vi "首页.vi"() -> ()   [LabVIEW 2016]
uses:
  <vilib>/Utility/miscctls.llb/LVPointTypeDef.ctl
  <vilib>/Utility/sysdir.llb/System Directory Type.ctl
  <vilib>/addons/database/_DB Variant To Data/Database Variant To Data.xnode
  PLC/PLC.lvlib
panel:
  out "大项目框 17":T1(xcontrol)
  out "大项目框 16":T1(xcontrol)
  out "大项目框 15":T1(xcontrol)
  out "大项目框 14":T1(xcontrol)
  out "大项目框 13":T1(xcontrol)
  in  "左箭头":bool
  in  "右箭头":bool
  out "大项目框 12":T1(xcontrol)
  out "大项目框 11":T1(xcontrol)
  out "大项目框 10":T1(xcontrol)
  out "大项目框 9":T1(xcontrol)
  out "大项目框 8":T1(xcontrol)
  out "大项目框 7":T1(xcontrol)
  out "大项目框 6":T1(xcontrol)
  out "大项目框 5":T1(xcontrol)
  out "大项目框 4":T1(xcontrol)
  out "大项目框 3":T1(xcontrol)
  out "大项目框 2":T1(xcontrol)
  out "大项目框":T1(xcontrol)
  out "湿度":string="75.5 %"
  out "室温":string="25.8 ℃"
  # "室温:"
  # "湿度:"
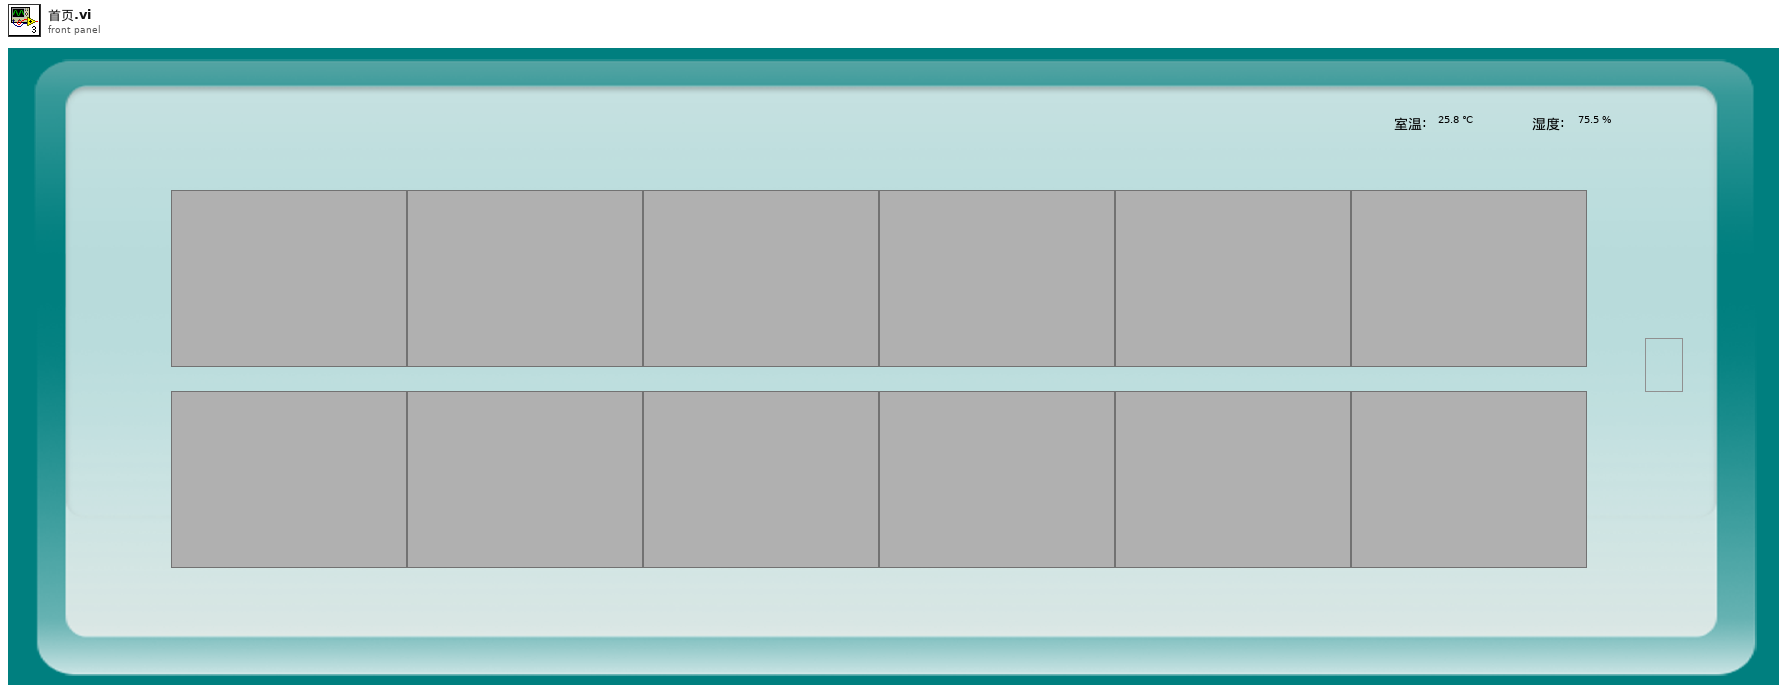
[diagram p1: front panel]
types:
  T1 = cluster{"中文项目名称":string, "英文项目名称":string, "单位":string, "浓度值":string}
  T2 = typedef "LVPointTypeDef.ctl" = cluster{"Horizontal":i16, "Vertical":i16}
  T3 = cluster{"AD0":sgl, "AD1":sgl, "AD2":sgl, "AD3":sgl, "AD4":sgl, "AD5":sgl}
  T4 = typedef "LVDateTimeRec.ctl" = cluster{"秒数的小数部分":dbl, "秒":i32, "分":i32, "时":i32, "日":i32, "月":i32, "年":i32, "天数（周）":i32, "天数（年）":i32, "DST":i32}
  T5 = cluster{"时间标识":timestamp, "监测值":sgl, "单位":string}
  T6 = cluster{"显示参数中文名":string, "显示参数英文名":string, "显示浓度":string, "显示单位":string}[]
  T7 = cluster{"显示参数中文名":string, "显示参数英文名":string, "显示浓度":string, "显示单位":string}
  T8 = typedef "System Directory Type.ctl" = i32
  T9 = cluster{"水温":bool, "pH":bool, "DO":bool, "Cond":bool, "Turb":bool, "氨氮":bool, "总磷":bool, "总氮":bool, "CODMn":bool, "CODCr":bool, "水位":bool, "流速":bool, "瞬时流量":bool, "室温":bool, "湿度":bool, "叶绿素a":bool, "藻密度":bool}
  T10 = cluster{"中文项目名称":string, "英文项目名称":string, "浓度值":string, "单位":string}
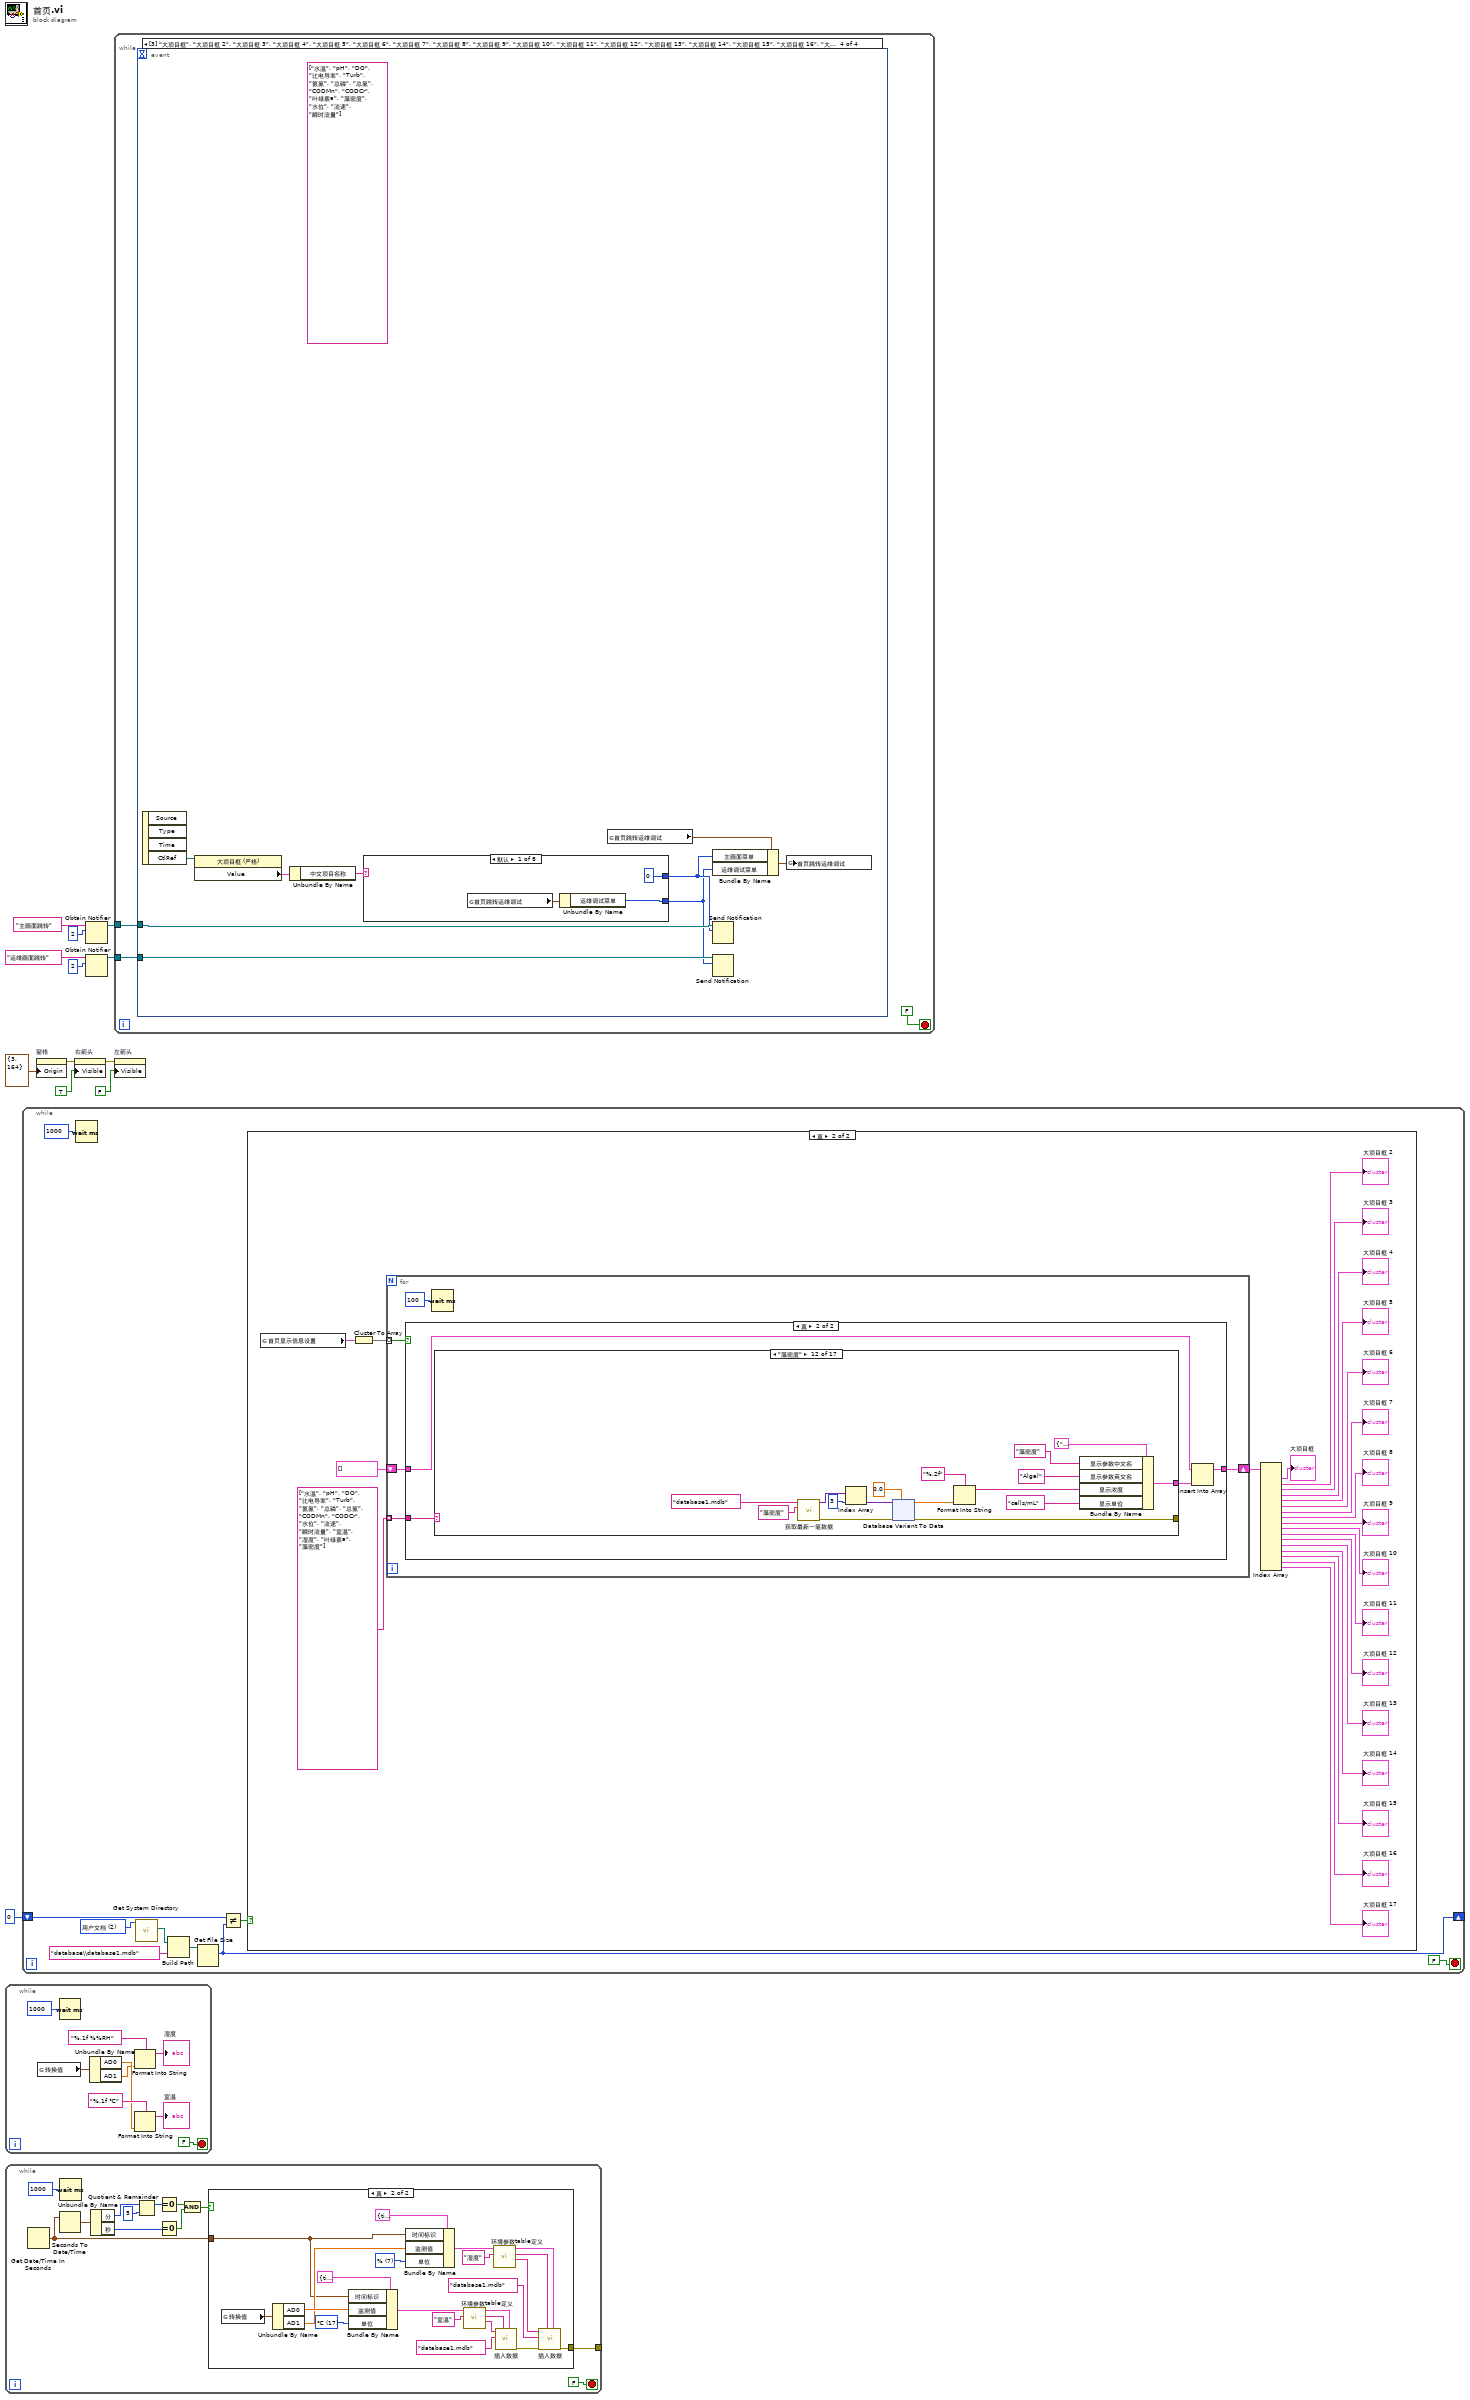
[diagram p0: block diagram]
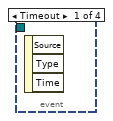
[diagram p3: hidden frame]
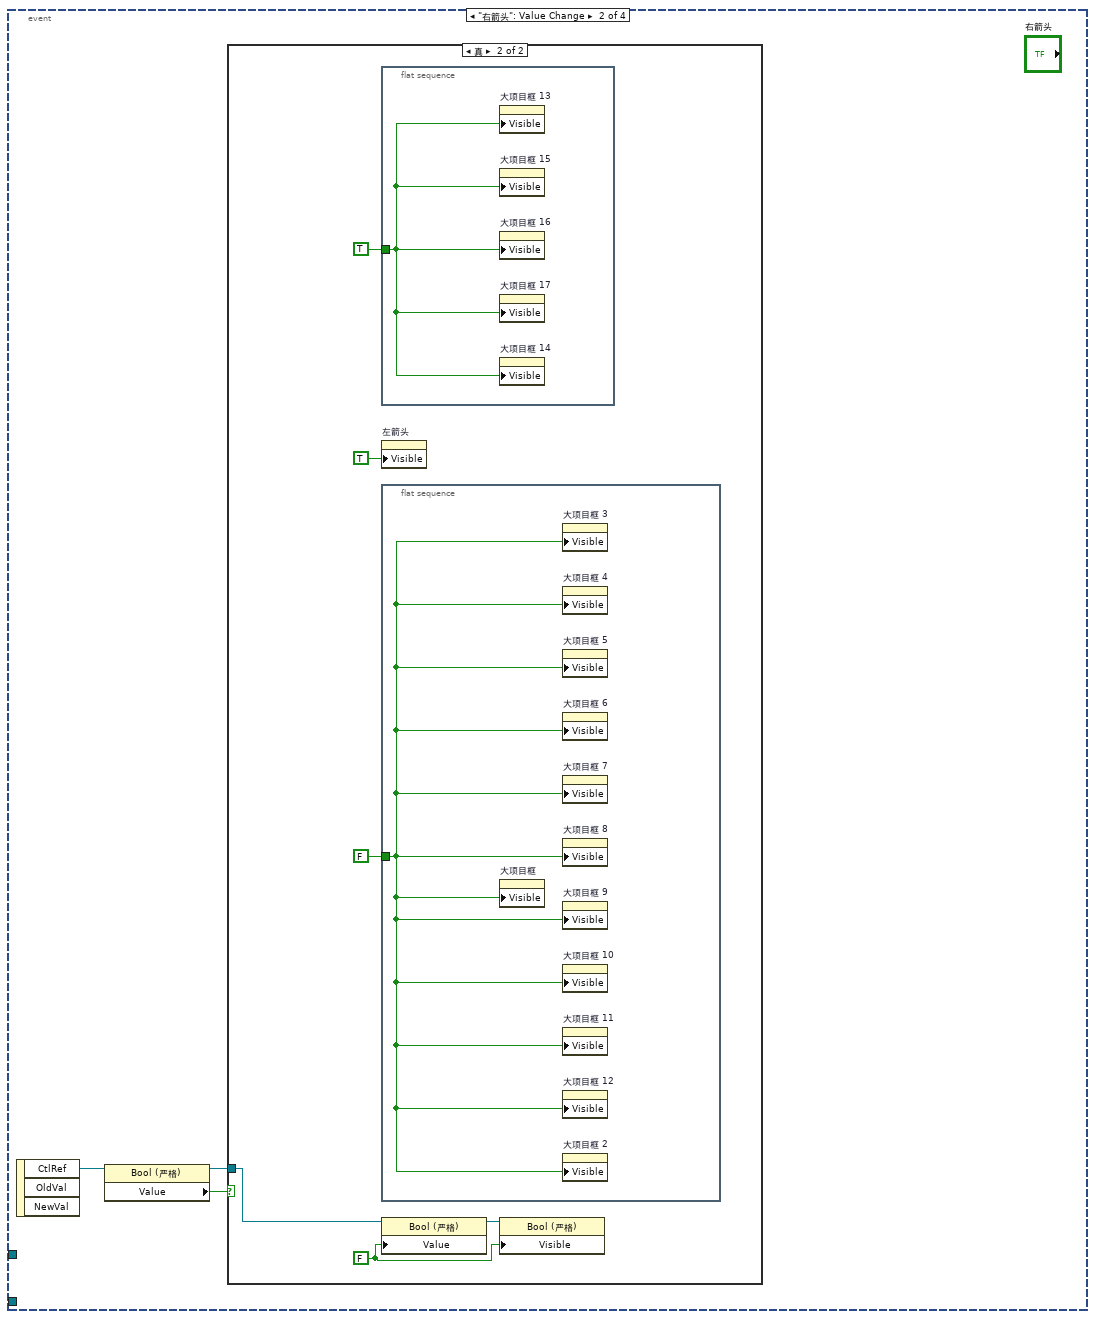
[diagram p4: hidden frame]
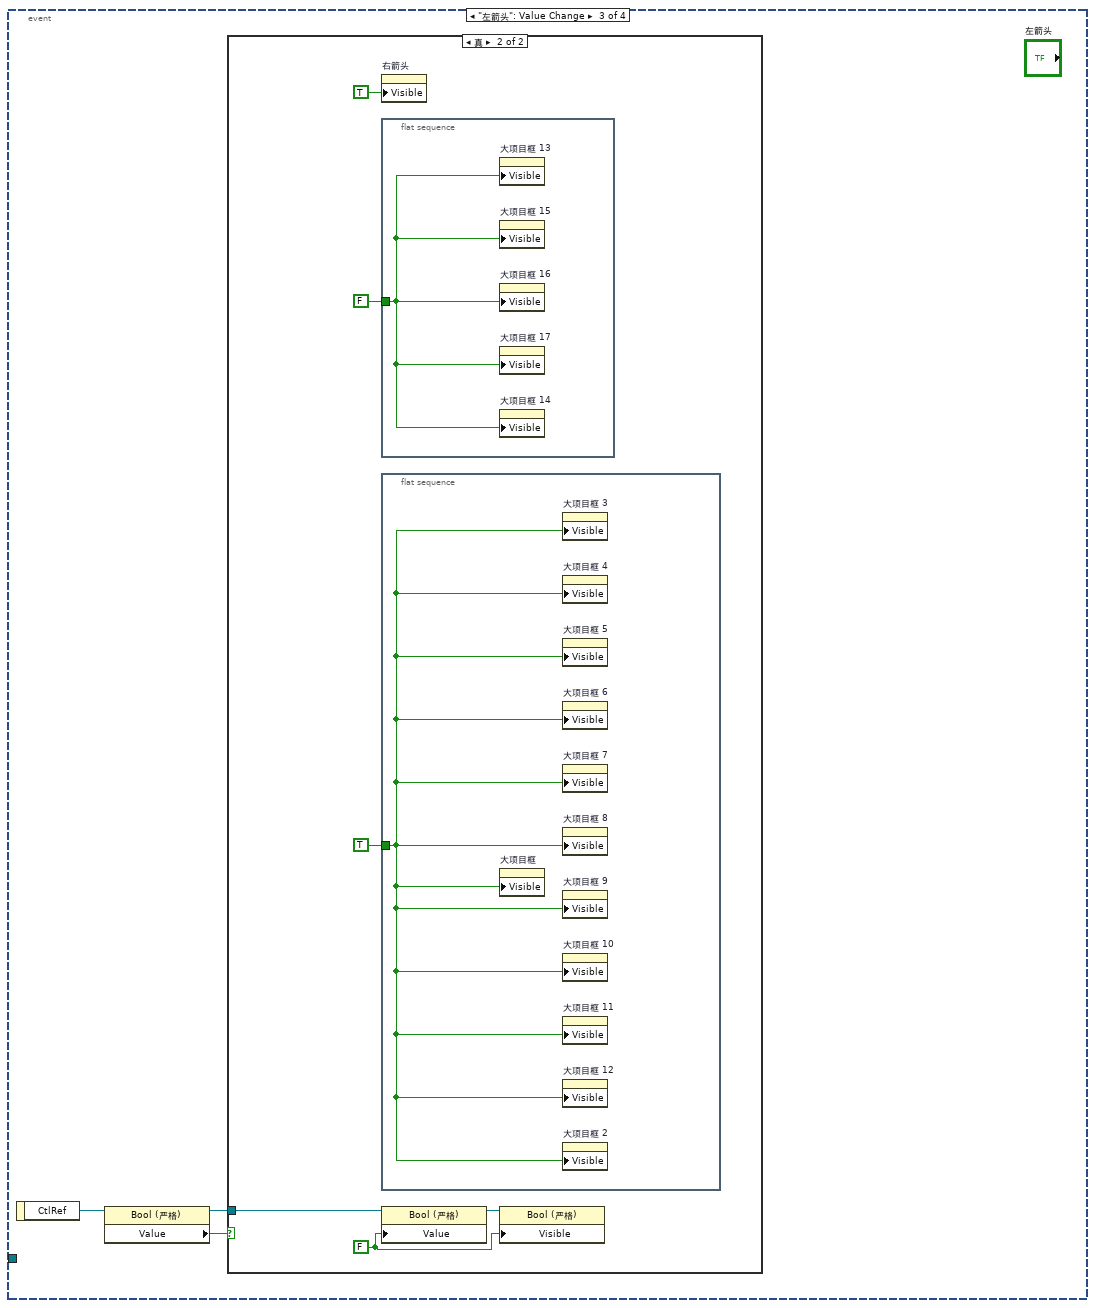
[diagram p6: hidden frame]
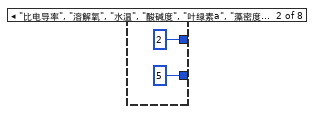
[diagram p8: hidden frame]
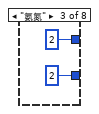
[diagram p9: hidden frame]
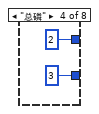
[diagram p10: hidden frame]
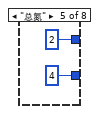
[diagram p11: hidden frame]
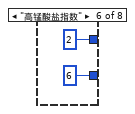
[diagram p12: hidden frame]
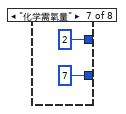
[diagram p13: hidden frame]
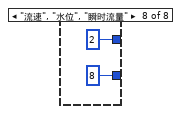
[diagram p14: hidden frame]
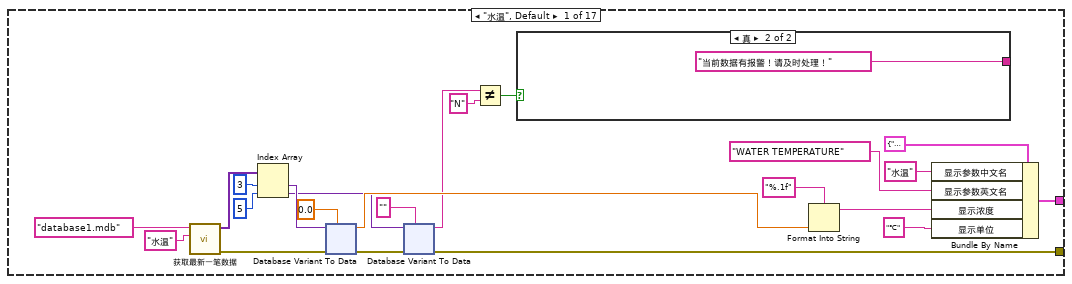
[diagram p17: hidden frame]
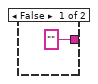
[diagram p18: hidden frame]
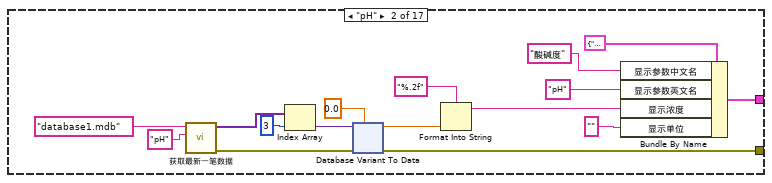
[diagram p19: hidden frame]
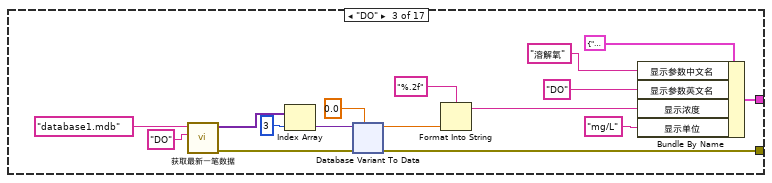
[diagram p20: hidden frame]
diagram:
  n1 = while {
    stop <- FALSE stop-if-true
    n2 = global read "采配水全局变量.vi" "转换值"() -> (w19:T3)
    n3 = Wait (ms)(milliseconds to wait=u32 1000 ("等待时间（毫秒）")) -> ()  [unwired: 1 out]
    n4 = Unbundle By Name(w19) -> ("AD0"=w14:sgl, "AD1"=w13:sgl)
    n5 = Format Into String(format string="%.1f %%RH" ("格式字符串"), w13) -> (resulting string=→"湿度":string)  [unwired: 2 in, 1 out]
    n6 = Format Into String(format string="%.1f ℃" ("格式字符串"), w14) -> (resulting string=→"室温":string)  [unwired: 2 in, 1 out]
  }
  n7 = while {
    tunnel: [w32] -> _
    stop <- FALSE stop-if-true
    n8 = Get Date/Time In Seconds() -> (seconds since 1Jan1904=w31:timestamp)
    n9 = Seconds To Date/Time(time stamp (now)=w31) -> (date time rec=w30:T4)  [unwired: 1 in]
    n10 = Wait (ms)(milliseconds to wait=u32 1000 ("等待时间（毫秒）")) -> ()  [unwired: 1 out]
    n11 = Unbundle By Name(w30) -> ("分"=w29:i32, "秒"=w27:i32)
    n12 = Quotient & Remainder(x=w29, y=5) -> (x-y*floor(x/y)=w26:i32)  [unwired: 1 out]
    n13 = Equal To 0?(x=w26) -> (x = 0?=w25:bool)
    n14 = Equal To 0?(x=w27) -> (x = 0?=w24:bool)
    n15 = Compound Arithmetic op=AND ("复合运算")(w25, w24) -> (w23:bool)
    n16 = case shown="真" w23 {
      tunnel: [_ w47] -> w32
      tunnel: w31 -> [_ w35]
      frame False {
      }
      frame True {
        w40 = u16 7 items=["ug/L", "mg/L", "ppm", "mg/m3", "cm", "ppb", "ug/m3", "%", "nmol/mol", "umol/mol", "MPN/L", "MPN/100ml", "ng/m3", "NTU", "无量纲", "ms/cm", "us/cm", "℃", "V"] ("单位")
        w44 = u16 17 items=["ug/L", "mg/L", "ppm", "mg/m3", "cm", "ppb", "ug/m3", "%", "nmol/mol", "umol/mol", "MPN/L", "MPN/100ml", "ng/m3", "NTU", "无量纲", "ms/cm", "us/cm", "℃", "V"] ("单位")
        n17 = global read "采配水全局变量.vi" "转换值"() -> (w55:T3)
        n18 = Unbundle By Name(w55) -> ("AD0"=w43:sgl, "AD1"=w41:sgl)
        n19 = Bundle By Name(cluster=cluster{"时间标识":timestamp, "监测值":sgl, "单位":u16} {"时间标识"=timestamp(0 s since 1904-01-01), "监测值"=0.0, "单位"=0} ("data"), "时间标识"=w35, "监测值"=w43, "单位"=w44) -> (w45:cluster{"时间标识":timestamp, "监测值":sgl, "单位":u16})
        n20 = Bundle By Name(cluster=cluster{"时间标识":timestamp, "监测值":sgl, "单位":u16} {"时间标识"=timestamp(0 s since 1904-01-01), "监测值"=0.0, "单位"=0} ("data"), "时间标识"=w35, "监测值"=w41, "单位"=w40) -> (w39:cluster{"时间标识":timestamp, "监测值":sgl, "单位":u16})
        n21 = call "环境参数table定义.vi"("table 输入"="室温", "data"=w45) -> ("table 输出"=w54:string, "columns"=w53:string[], "data输出"=w52:T5)  [unwired: 7 in]
        n22 = call "环境参数table定义.vi"("table 输入"="湿度", "data"=w39) -> ("table 输出"=w49:string, "columns"=w50:string[], "data输出"=w51:T5)  [unwired: 7 in]
        n23 = call "插入数据.vi"("data"=w52, "columns"=w53, "database"="database1.mdb" ("table 输入"), "table"=w54) -> ("error out"=w48:errorcluster)  [unwired: 7 in]
        n24 = call "插入数据.vi"("data"=w51, "columns"=w50, "error in (no error)"=w48, "database"="database1.mdb" ("table 输入"), "table"=w49) -> ("error out"=w47:errorcluster)  [unwired: 6 in]
      }
    }
  }
  n25 = while {
    shift-right: [w57] -> _
    shift-left: i64 0 ("大小（字节）") -> [w58]
    stop <- FALSE stop-if-true
    w62 = T8 2 items=["用户目录"=0, "用户桌面"=1, "用户文档"=2, "用户应用程序数据"=3, "用户设置"=4, "用户临时目录"=5, "公共文档"=6, "公共应用程序数据"=7, "公共设置"=8, "公共缓存"=13, "系统核心库"=9, "系统安装库"=10, "应用程序文件"=11, "启动盘根目录"=12] ("system directory type")
    n26 = Wait (ms)(milliseconds to wait=u32 1000 ("等待时间（毫秒）")) -> ()  [unwired: 1 out]
    n27 = call <vilib>:"Get System Directory.vi"("system directory type"=w62) -> ("system directory"=w61:path)  [unwired: 10 in]
    n28 = Build Path(base path=w61, name or relative path="database\\database1.mdb" ("名称或相对路径")) -> (appended path=w60:path)
    n29 = Get File Size(file=w60) -> (size (in bytes)=w57:i64)  [unwired: 1 in, 2 out]
    n30 = Not Equal?(x=w58, y=w57) -> (x != y?=w56:bool)
    n31 = case shown="真" w56 {
      frame False {
      }
      frame True {
        n32 = global read "系统设置全局变量.vi" "首页显示信息设置"() -> (w66:T9)
        n33 = Cluster To Array(cluster=w66) -> (array=w65:bool[])
        n34 = for {
          tunnel: w65 -> [w91] mode=indexing
          tunnel: string[] ["水温", "pH", "DO", "比电导率", "Turb", "氨氮", "总磷", "总氮", "CODMn", "CODCr", "水位", "流速", "瞬时流量", "室温", "湿度", "叶绿素a", "藻密度"] -> [w90] mode=indexing
          shift-right: [w88] -> w86
          shift-left: T6 [] -> [w89]
          n35 = case shown="真" w91 {
            tunnel: w90 -> [_ w96]
            tunnel: w89 -> [w92 w95]
            tunnel: [w92 w94] -> w88
            frame False {
            }
            frame True {
              n36 = case shown="\"藻密度\"" w96 {
                tunnel: [w105 w197 w245 w293 w341 w389 w437 w485 w533 w581 w619 w667 w717 w725 w730 w740 w749] -> w93
                tunnel: [w97 w186 w234 w282 w330 w378 w426 w474 w522 w570 w618 w666 _ _ _ _ _] -> _
                frame "水温", Default {
                  n37 = call "获取最新一笔数据.vi"("table"="水温", "database"="database1.mdb" ("名称或相对路径")) -> ("error out"=w106:errorcluster, "子数组"=w112:variant[])  [unwired: 8 in]
                  n38 = Index Array(array=w112, index #1=3 ("索引"), index #2=5 ("索引")) -> (element #1=w110:variant, element #2=w102:variant)
                  n39 = xnode "Database Variant To Data"("database variant"=w110, "error in (no error)"=w106, "type"=0.0) -> ("data"=w107:dbl, "error out"=w98:errorcluster)
                  n40 = xnode "Database Variant To Data"("database variant"=w102, "error in (no error)"=w98, "type"="") -> ("data"=w101:string, "error out"=w97:errorcluster)
                  n41 = Not Equal?(x=w101, y="N") -> (x != y?=w99:bool)
                  n42 = case shown="真" w99 {
                    tunnel: ["" "当前数据有报警！请及时处理！" ("y")] -> _
                    frame False {
                    }
                    frame True {
                    }
                  }
                  n43 = Format Into String(format string="%.1f" ("格式字符串"), w107) -> (resulting string=w114:string)  [unwired: 2 in, 1 out]
                  n44 = Bundle By Name(cluster=T7 {"显示参数中文名"="", "显示参数英文名"="", "显示浓度"="", "显示单位"=""} ("元素"), "显示参数中文名"="水温", "显示参数英文名"="WATER TEMPERATURE", "显示浓度"=w114, "显示单位"="℃") -> (w105:T7)
                }
                frame "pH" {
                  n45 = call "获取最新一笔数据.vi"("table"="pH", "database"="database1.mdb" ("名称或相对路径")) -> ("error out"=w187:errorcluster, "子数组"=w193:variant[])  [unwired: 8 in]
                  n46 = Index Array(array=w193, index=3 ("索引")) -> (element=w191:variant)
                  n47 = xnode "Database Variant To Data"("database variant"=w191, "error in (no error)"=w187, "type"=0.0) -> ("data"=w188:dbl, "error out"=w186:errorcluster)
                  n48 = Format Into String(format string="%.2f" ("格式字符串"), w188) -> (resulting string=w195:string)  [unwired: 2 in, 1 out]
                  n49 = Bundle By Name(cluster=T7 {"显示参数中文名"="", "显示参数英文名"="", "显示浓度"="", "显示单位"=""} ("元素"), "显示参数中文名"="酸碱度", "显示参数英文名"="pH", "显示浓度"=w195, "显示单位"="") -> (w197:T7)
                }
                frame "DO" {
                  n50 = call "获取最新一笔数据.vi"("table"="DO", "database"="database1.mdb" ("名称或相对路径")) -> ("error out"=w235:errorcluster, "子数组"=w241:variant[])  [unwired: 8 in]
                  n51 = Index Array(array=w241, index=3 ("索引")) -> (element=w239:variant)
                  n52 = xnode "Database Variant To Data"("database variant"=w239, "error in (no error)"=w235, "type"=0.0) -> ("data"=w236:dbl, "error out"=w234:errorcluster)
                  n53 = Format Into String(format string="%.2f" ("格式字符串"), w236) -> (resulting string=w243:string)  [unwired: 2 in, 1 out]
                  n54 = Bundle By Name(cluster=T7 {"显示参数中文名"="", "显示参数英文名"="", "显示浓度"="", "显示单位"=""} ("元素"), "显示参数中文名"="溶解氧", "显示参数英文名"="DO", "显示浓度"=w243, "显示单位"="mg/L") -> (w245:T7)
                }
                frame "比电导率" {
                  n55 = call "获取最新一笔数据.vi"("table"="比电导率", "database"="database1.mdb" ("名称或相对路径")) -> ("error out"=w283:errorcluster, "子数组"=w289:variant[])  [unwired: 8 in]
                  n56 = Index Array(array=w289, index=3 ("索引")) -> (element=w287:variant)
                  n57 = xnode "Database Variant To Data"("database variant"=w287, "error in (no error)"=w283, "type"=0.0) -> ("data"=w284:dbl, "error out"=w282:errorcluster)
                  n58 = Format Into String(format string="%.1f" ("格式字符串"), w284) -> (resulting string=w291:string)  [unwired: 2 in, 1 out]
                  n59 = Bundle By Name(cluster=T7 {"显示参数中文名"="", "显示参数英文名"="", "显示浓度"="", "显示单位"=""} ("元素"), "显示参数中文名"="比电导率", "显示参数英文名"="spCond", "显示浓度"=w291, "显示单位"="μS/cm") -> (w293:T7)
                }
                frame "Turb" {
                  n60 = call "获取最新一笔数据.vi"("table"="浊度", "database"="database1.mdb" ("名称或相对路径")) -> ("error out"=w331:errorcluster, "子数组"=w337:variant[])  [unwired: 8 in]
                  n61 = Index Array(array=w337, index=3 ("索引")) -> (element=w335:variant)
                  n62 = xnode "Database Variant To Data"("database variant"=w335, "error in (no error)"=w331, "type"=0.0) -> ("data"=w332:dbl, "error out"=w330:errorcluster)
                  n63 = Format Into String(format string="%.1f" ("格式字符串"), w332) -> (resulting string=w339:string)  [unwired: 2 in, 1 out]
                  n64 = Bundle By Name(cluster=T7 {"显示参数中文名"="", "显示参数英文名"="", "显示浓度"="", "显示单位"=""} ("元素"), "显示参数中文名"="浊度", "显示参数英文名"="Turb", "显示浓度"=w339, "显示单位"="NTU") -> (w341:T7)
                }
                frame "氨氮" {
                  n65 = call "获取最新一笔数据.vi"("table"="氨氮", "database"="database1.mdb" ("名称或相对路径")) -> ("error out"=w379:errorcluster, "子数组"=w385:variant[])  [unwired: 8 in]
                  n66 = Index Array(array=w385, index=3 ("索引")) -> (element=w383:variant)
                  n67 = xnode "Database Variant To Data"("database variant"=w383, "error in (no error)"=w379, "type"=0.0) -> ("data"=w380:dbl, "error out"=w378:errorcluster)
                  n68 = Format Into String(format string="%.3f" ("格式字符串"), w380) -> (resulting string=w387:string)  [unwired: 2 in, 1 out]
                  n69 = Bundle By Name(cluster=T7 {"显示参数中文名"="", "显示参数英文名"="", "显示浓度"="", "显示单位"=""} ("元素"), "显示参数中文名"="氨氮", "显示参数英文名"="NPA", "显示浓度"=w387, "显示单位"="mg/L") -> (w389:T7)
                }
                frame "总磷" {
                  n70 = call "获取最新一笔数据.vi"("table"="总磷", "database"="database1.mdb" ("名称或相对路径")) -> ("error out"=w427:errorcluster, "子数组"=w433:variant[])  [unwired: 8 in]
                  n71 = Index Array(array=w433, index=3 ("索引")) -> (element=w431:variant)
                  n72 = xnode "Database Variant To Data"("database variant"=w431, "error in (no error)"=w427, "type"=0.0) -> ("data"=w428:dbl, "error out"=w426:errorcluster)
                  n73 = Format Into String(format string="%.3f" ("格式字符串"), w428) -> (resulting string=w435:string)  [unwired: 2 in, 1 out]
                  n74 = Bundle By Name(cluster=T7 {"显示参数中文名"="", "显示参数英文名"="", "显示浓度"="", "显示单位"=""} ("元素"), "显示参数中文名"="总磷", "显示参数英文名"="TP", "显示浓度"=w435, "显示单位"="mg/L") -> (w437:T7)
                }
                frame "总氮" {
                  n75 = call "获取最新一笔数据.vi"("table"="总氮", "database"="database1.mdb" ("名称或相对路径")) -> ("error out"=w475:errorcluster, "子数组"=w481:variant[])  [unwired: 8 in]
                  n76 = Index Array(array=w481, index=3 ("索引")) -> (element=w479:variant)
                  n77 = xnode "Database Variant To Data"("database variant"=w479, "error in (no error)"=w475, "type"=0.0) -> ("data"=w476:dbl, "error out"=w474:errorcluster)
                  n78 = Format Into String(format string="%.2f" ("格式字符串"), w476) -> (resulting string=w483:string)  [unwired: 2 in, 1 out]
                  n79 = Bundle By Name(cluster=T7 {"显示参数中文名"="", "显示参数英文名"="", "显示浓度"="", "显示单位"=""} ("元素"), "显示参数中文名"="总氮", "显示参数英文名"="TN", "显示浓度"=w483, "显示单位"="mg/L") -> (w485:T7)
                }
                frame "CODMn" {
                  n80 = call "获取最新一笔数据.vi"("table"="CODmn", "database"="database1.mdb" ("名称或相对路径")) -> ("error out"=w523:errorcluster, "子数组"=w529:variant[])  [unwired: 8 in]
                  n81 = Index Array(array=w529, index=3 ("索引")) -> (element=w527:variant)
                  n82 = xnode "Database Variant To Data"("database variant"=w527, "error in (no error)"=w523, "type"=0.0) -> ("data"=w524:dbl, "error out"=w522:errorcluster)
                  n83 = Format Into String(format string="%.2f" ("格式字符串"), w524) -> (resulting string=w531:string)  [unwired: 2 in, 1 out]
                  n84 = Bundle By Name(cluster=T7 {"显示参数中文名"="", "显示参数英文名"="", "显示浓度"="", "显示单位"=""} ("元素"), "显示参数中文名"="高锰酸盐指数", "显示参数英文名"="CODmn", "显示浓度"=w531, "显示单位"="mg/L") -> (w533:T7)
                }
                frame "CODCr" {
                  n85 = call "获取最新一笔数据.vi"("table"="CODCr", "database"="database1.mdb" ("名称或相对路径")) -> ("error out"=w571:errorcluster, "子数组"=w577:variant[])  [unwired: 8 in]
                  n86 = Index Array(array=w577, index=3 ("索引")) -> (element=w575:variant)
                  n87 = xnode "Database Variant To Data"("database variant"=w575, "error in (no error)"=w571, "type"=0.0) -> ("data"=w572:dbl, "error out"=w570:errorcluster)
                  n88 = Format Into String(format string="%.2f" ("格式字符串"), w572) -> (resulting string=w579:string)  [unwired: 2 in, 1 out]
                  n89 = Bundle By Name(cluster=T7 {"显示参数中文名"="", "显示参数英文名"="", "显示浓度"="", "显示单位"=""} ("元素"), "显示参数中文名"="化学需氧量", "显示参数英文名"="CODCr", "显示浓度"=w579, "显示单位"="mg/L") -> (w581:T7)
                }
                frame "叶绿素a" {
                  n90 = call "获取最新一笔数据.vi"("table"="叶绿素a", "database"="database1.mdb" ("名称或相对路径")) -> ("error out"=w620:errorcluster, "子数组"=w626:variant[])  [unwired: 8 in]
                  n91 = Index Array(array=w626, index=3 ("索引")) -> (element=w624:variant)
                  n92 = xnode "Database Variant To Data"("database variant"=w624, "error in (no error)"=w620, "type"=0.0) -> ("data"=w621:dbl, "error out"=w618:errorcluster)
                  n93 = Format Into String(format string="%.2f" ("格式字符串"), w621) -> (resulting string=w628:string)  [unwired: 2 in, 1 out]
                  n94 = Bundle By Name(cluster=T7 {"显示参数中文名"="", "显示参数英文名"="", "显示浓度"="", "显示单位"=""} ("元素"), "显示参数中文名"="叶绿素a", "显示参数英文名"="Chla", "显示浓度"=w628, "显示单位"="μg/L") -> (w619:T7)
                }
                frame "藻密度" {
                  n95 = call "获取最新一笔数据.vi"("table"="藻密度", "database"="database1.mdb" ("名称或相对路径")) -> ("error out"=w668:errorcluster, "子数组"=w674:variant[])  [unwired: 8 in]
                  n96 = Index Array(array=w674, index=3 ("索引")) -> (element=w672:variant)
                  n97 = xnode "Database Variant To Data"("database variant"=w672, "error in (no error)"=w668, "type"=0.0) -> ("data"=w669:dbl, "error out"=w666:errorcluster)
                  n98 = Format Into String(format string="%.2f" ("格式字符串"), w669) -> (resulting string=w676:string)  [unwired: 2 in, 1 out]
                  n99 = Bundle By Name(cluster=T7 {"显示参数中文名"="", "显示参数英文名"="", "显示浓度"="", "显示单位"=""} ("元素"), "显示参数中文名"="藻密度", "显示参数英文名"="Algal", "显示浓度"=w676, "显示单位"="cells/mL") -> (w667:T7)
                }
                frame "水位" {
                  n100 = global read "流量计全局变量.vi" "水位"() -> (w714:dbl)
                  n101 = Format Into String(format string="%.2f" ("格式字符串"), w714) -> (resulting string=w715:string)  [unwired: 2 in, 1 out]
                  n102 = Bundle By Name(cluster=T7 {"显示参数中文名"="", "显示参数英文名"="", "显示浓度"="", "显示单位"=""} ("元素"), "显示参数中文名"="水位", "显示参数英文名"="WaterLevel", "显示浓度"=w715, "显示单位"="m") -> (w717:T7)
                }
                frame "流速" {
                  n103 = global read "流量计全局变量.vi" "瞬时流速"() -> (w722:dbl)
                  n104 = Format Into String(format string="%.2f" ("格式字符串"), w722) -> (resulting string=w723:string)  [unwired: 2 in, 1 out]
                  n105 = Bundle By Name(cluster=T7 {"显示参数中文名"="", "显示参数英文名"="", "显示浓度"="", "显示单位"=""} ("元素"), "显示参数中文名"="流速", "显示参数英文名"="FlowRate", "显示浓度"=w723, "显示单位"="m/s") -> (w725:T7)
                }
                frame "瞬时流量" {
                  n106 = global read "流量计全局变量.vi" "瞬时流量"() -> (w731:dbl)
                  n107 = Format Into String(format string="%.2f" ("格式字符串"), w731) -> (resulting string=w732:string)  [unwired: 2 in, 1 out]
                  n108 = Bundle By Name(cluster=T7 {"显示参数中文名"="", "显示参数英文名"="", "显示浓度"="", "显示单位"=""} ("元素"), "显示参数中文名"="瞬时流量", "显示参数英文名"="InstantaneousFlow", "显示浓度"=w732, "显示单位"="m3/s") -> (w730:T7)
                }
                frame "室温" {
                  n109 = global read "采配水全局变量.vi" "转换值"() -> (w739:T3)
                  n110 = Unbundle By Name(w739) -> ("AD0"=w738:sgl)
                  n111 = Format Into String(format string="%.2f" ("格式字符串"), w738) -> (resulting string=w741:string)  [unwired: 2 in, 1 out]
                  n112 = Bundle By Name(cluster=T7 {"显示参数中文名"="", "显示参数英文名"="", "显示浓度"="", "显示单位"=""} ("元素"), "显示参数中文名"="室温", "显示参数英文名"="Room Temperature ", "显示浓度"=w741, "显示单位"="℃") -> (w740:T7)
                }
                frame "湿度" {
                  n113 = global read "采配水全局变量.vi" "转换值"() -> (w748:T3)
                  n114 = Unbundle By Name(w748) -> ("AD1"=w747:sgl)
                  n115 = Format Into String(format string="%.2f" ("格式字符串"), w747) -> (resulting string=w750:string)  [unwired: 2 in, 1 out]
                  n116 = Bundle By Name(cluster=T7 {"显示参数中文名"="", "显示参数英文名"="", "显示浓度"="", "显示单位"=""} ("元素"), "显示参数中文名"="相对湿度", "显示参数英文名"="Relative Humidity", "显示浓度"=w750, "显示单位"="%RH") -> (w749:T7)
                }
              }
              n117 = Insert Into Array(array=w95, new element=w93) -> (w94:T6)  [unwired: 1 in]
            }
          }
          n118 = Wait (ms)(milliseconds to wait=u32 100 ("等待时间（毫秒）")) -> ()  [unwired: 1 out]
        }
        n119 = Index Array(array=w86) -> (element #1=→"大项目框":T7, element #2=→"大项目框 2":T7, element #3=→"大项目框 3":T7, element #4=→"大项目框 4":T7, element #5=→"大项目框 5":T7, element #6=→"大项目框 6":T7, element #7=→"大项目框 7":T7, element #8=→"大项目框 8":T7, element #9=→"大项目框 9":T7, element #10=→"大项目框 10":T7, element #11=→"大项目框 11":T7, element #12=→"大项目框 12":T7, element #13=→"大项目框 13":T7, element #14=→"大项目框 14":T7, element #15=→"大项目框 15":T7, element #16=→"大项目框 16":T7, element #17=→"大项目框 17":T7)  [unwired: 17 in]
      }
    }
  }
  n120 = property on="窗格" class="Pane"("Origin"=T2 {"Horizontal"=3, "Vertical"=164} ("原点")) -> (error out=w9:errorcluster)  [unwired: 2 in, 1 out]
  n121 = property on="右箭头" class="Bool (严格)"(error in=w9, "Visible"=TRUE ("可见")) -> (error out=w8:errorcluster)  [unwired: 1 in, 1 out]
  n122 = Obtain Notifier(name (unnamed)="主画面跳转" ("名称（未命名）"), notification data type=2 ("主画面菜单")) -> (notifier out=w7:refnum<notifier>)  [unwired: 2 in, 2 out]
  n123 = Obtain Notifier(name (unnamed)="运维画面跳转" ("名称（未命名）"), notification data type=2 ("主画面菜单")) -> (notifier out=w2:refnum<notifier>)  [unwired: 2 in, 2 out]
  n124 = property on="左箭头" class="Bool (严格)"(error in=w8, "Visible"=FALSE ("可见")) -> ()  [unwired: 1 in, 2 out]
  n125 = while {
    tunnel: w7 -> [w757]
    tunnel: w2 -> [w756]
    stop <- FALSE stop-if-true
    n126 = event shown="[3] \"大项目框\", \"大项目框 2\", \"大项目框 3\", \"大项目框 4\", \"大项目框 5\", \"大项目框 6\", \"大项目框 7\", \"大项目框 8\", \"大项目框 9\", \"大项目框 10\", \"大项目框 11\", \"大项目框 12\", \"大项目框 13\", \"大项目框 14\", \"大项目框 15\", \"大项目框 16\", \"大项目框 17\": 鼠标按下" {
      selector: _ -> [_ _ _ _]
      dyn-events: _ -> [_ _ _ _]
      timeout: _ -> [_ _ _ _]
      tunnel: w757 -> [_ _ _ w785]
      tunnel: w756 -> [_ _ _ w782]
      event Timeout {
        n127 = event-data() -> ()  [unwired: 1 in, 3 out]
      }
      event "右箭头": Value Change {
        n128 = event-data() -> ("CtlRef"=w761:refnum<vi>)  [unwired: 1 in, 2 out]
        n129 = property class="Bool (严格)"(reference=w761) -> (reference out=w759:refnum<vi>, "Value"=w760:bool)  [unwired: 1 in, 1 out]
        n130 = case shown="真" w760 {
          tunnel: w759 -> [_ w767]
          frame False {
          }
          frame True {
            w766 = FALSE ("值")
            n131 = flat-sequence {
              tunnel: TRUE ("可见") -> [w768]
              frame #0 {
                n132 = property on="大项目框 13" class="大项目框 (严格)"("Visible"=w768) -> ()  [unwired: 2 in, 2 out]
                n133 = property on="大项目框 15" class="大项目框 (严格)"("Visible"=w768) -> ()  [unwired: 2 in, 2 out]
                n134 = property on="大项目框 16" class="大项目框 (严格)"("Visible"=w768) -> ()  [unwired: 2 in, 2 out]
                n135 = property on="大项目框 17" class="大项目框 (严格)"("Visible"=w768) -> ()  [unwired: 2 in, 2 out]
                n136 = property on="大项目框 14" class="大项目框 (严格)"("Visible"=w768) -> ()  [unwired: 2 in, 2 out]
              }
            }
            n137 = property on="左箭头" class="Bool (严格)"("Visible"=TRUE ("可见")) -> ()  [unwired: 2 in, 2 out]
            n138 = flat-sequence {
              tunnel: FALSE ("可见") -> [w769]
              frame #0 {
                n139 = property on="大项目框" class="大项目框 (严格)"("Visible"=w769) -> ()  [unwired: 2 in, 2 out]
                n140 = property on="大项目框 3" class="大项目框 (严格)"("Visible"=w769) -> ()  [unwired: 2 in, 2 out]
                n141 = property on="大项目框 4" class="大项目框 (严格)"("Visible"=w769) -> ()  [unwired: 2 in, 2 out]
                n142 = property on="大项目框 5" class="大项目框 (严格)"("Visible"=w769) -> ()  [unwired: 2 in, 2 out]
                n143 = property on="大项目框 6" class="大项目框 (严格)"("Visible"=w769) -> ()  [unwired: 2 in, 2 out]
                n144 = property on="大项目框 7" class="大项目框 (严格)"("Visible"=w769) -> ()  [unwired: 2 in, 2 out]
                n145 = property on="大项目框 8" class="大项目框 (严格)"("Visible"=w769) -> ()  [unwired: 2 in, 2 out]
                n146 = property on="大项目框 9" class="大项目框 (严格)"("Visible"=w769) -> ()  [unwired: 2 in, 2 out]
                n147 = property on="大项目框 10" class="大项目框 (严格)"("Visible"=w769) -> ()  [unwired: 2 in, 2 out]
                n148 = property on="大项目框 11" class="大项目框 (严格)"("Visible"=w769) -> ()  [unwired: 2 in, 2 out]
                n149 = property on="大项目框 12" class="大项目框 (严格)"("Visible"=w769) -> ()  [unwired: 2 in, 2 out]
                n150 = property on="大项目框 2" class="大项目框 (严格)"("Visible"=w769) -> ()  [unwired: 2 in, 2 out]
              }
            }
            n151 = property class="Bool (严格)"(reference=w767, "Value"=w766) -> (reference out=w765:refnum<vi>)  [unwired: 1 in, 1 out]
            n152 = property class="Bool (严格)"(reference=w765, "Visible"=w766) -> ()  [unwired: 1 in, 2 out]
          }
        }
      }
      event "左箭头": Value Change {
        n153 = event-data() -> ("CtlRef"=w772:refnum<vi>)  [unwired: 1 in]
        n154 = property class="Bool (严格)"(reference=w772) -> (reference out=w770:refnum<vi>, "Value"=w771:bool)  [unwired: 1 in, 1 out]
        n155 = case shown="真" w771 {
          tunnel: w770 -> [_ w778]
          frame False {
          }
          frame True {
            w777 = FALSE ("值")
            n156 = property on="右箭头" class="Bool (严格)"("Visible"=TRUE ("可见")) -> ()  [unwired: 2 in, 2 out]
            n157 = flat-sequence {
              tunnel: FALSE ("可见") -> [w779]
              frame #0 {
                n158 = property on="大项目框 13" class="大项目框 (严格)"("Visible"=w779) -> ()  [unwired: 2 in, 2 out]
                n159 = property on="大项目框 15" class="大项目框 (严格)"("Visible"=w779) -> ()  [unwired: 2 in, 2 out]
                n160 = property on="大项目框 16" class="大项目框 (严格)"("Visible"=w779) -> ()  [unwired: 2 in, 2 out]
                n161 = property on="大项目框 17" class="大项目框 (严格)"("Visible"=w779) -> ()  [unwired: 2 in, 2 out]
                n162 = property on="大项目框 14" class="大项目框 (严格)"("Visible"=w779) -> ()  [unwired: 2 in, 2 out]
              }
            }
            n163 = flat-sequence {
              tunnel: TRUE ("可见") -> [w780]
              frame #0 {
                n164 = property on="大项目框" class="大项目框 (严格)"("Visible"=w780) -> ()  [unwired: 2 in, 2 out]
                n165 = property on="大项目框 3" class="大项目框 (严格)"("Visible"=w780) -> ()  [unwired: 2 in, 2 out]
                n166 = property on="大项目框 4" class="大项目框 (严格)"("Visible"=w780) -> ()  [unwired: 2 in, 2 out]
                n167 = property on="大项目框 5" class="大项目框 (严格)"("Visible"=w780) -> ()  [unwired: 2 in, 2 out]
                n168 = property on="大项目框 6" class="大项目框 (严格)"("Visible"=w780) -> ()  [unwired: 2 in, 2 out]
                n169 = property on="大项目框 7" class="大项目框 (严格)"("Visible"=w780) -> ()  [unwired: 2 in, 2 out]
                n170 = property on="大项目框 8" class="大项目框 (严格)"("Visible"=w780) -> ()  [unwired: 2 in, 2 out]
                n171 = property on="大项目框 9" class="大项目框 (严格)"("Visible"=w780) -> ()  [unwired: 2 in, 2 out]
                n172 = property on="大项目框 10" class="大项目框 (严格)"("Visible"=w780) -> ()  [unwired: 2 in, 2 out]
                n173 = property on="大项目框 11" class="大项目框 (严格)"("Visible"=w780) -> ()  [unwired: 2 in, 2 out]
                n174 = property on="大项目框 12" class="大项目框 (严格)"("Visible"=w780) -> ()  [unwired: 2 in, 2 out]
                n175 = property on="大项目框 2" class="大项目框 (严格)"("Visible"=w780) -> ()  [unwired: 2 in, 2 out]
              }
            }
            n176 = property class="Bool (严格)"(reference=w778, "Value"=w777) -> (reference out=w776:refnum<vi>)  [unwired: 1 in, 1 out]
            n177 = property class="Bool (严格)"(reference=w776, "Visible"=w777) -> ()  [unwired: 1 in, 2 out]
          }
        }
      }
      event "大项目框", "大项目框 2", "大项目框 3", "大项目框 4", "大项目框 5", "大项目框 6", "大项目框 7", "大项目框 8", "大项目框 9", "大项目框 10", "大项目框 11", "大项目框 12", "大项目框 13", "大项目框 14", "大项目框 15", "大项目框 16", "大项目框 17": Mouse Down {
        (unwired) string[] ["水温", "pH", "DO", "比电导率", "Turb", "氨氮", "总磷", "总氮", "CODMn", "CODCr", "叶绿素a", "藻密度", "水位", "流速", "瞬时流量"]
        n178 = event-data() -> ("CtlRef"=w789:refnum<vi>)  [unwired: 1 in, 3 out]
        n179 = property class="大项目框 (严格)"(reference=w789) -> ("Value"=w788:T10)  [unwired: 1 in, 2 out]
        n180 = Unbundle By Name(w788) -> ("中文项目名称"=w787:string)
        n181 = case shown="默认" w787 {
          tunnel: [w791 5 ("运维调试菜单") 2 ("运维调试菜单") 3 ("运维调试菜单") 4 ("运维调试菜单") 6 ("运维调试菜单") 7 ("运维调试菜单") 8 ("运维调试菜单")] -> w781
          tunnel: [0 ("运维调试菜单") 2 ("运维调试菜单") 2 ("运维调试菜单") 2 ("运维调试菜单") 2 ("运维调试菜单") 2 ("运维调试菜单") 2 ("运维调试菜单") 2 ("运维调试菜单")] -> w783
          frame Default {
            n182 = global read "系统设置全局变量.vi" "首页跳转运维调试"() -> (w792:cluster{"主画面菜单":i32, "运维调试菜单":i32})
            n183 = Unbundle By Name(w792) -> ("运维调试菜单"=w791:i32)
          }
          frame "比电导率", "溶解氧", "水温", "酸碱度", "叶绿素a", "藻密度", "浊度" {
          }
          frame "氨氮" {
          }
          frame "总磷" {
          }
          frame "总氮" {
          }
          frame "高锰酸盐指数" {
          }
          frame "化学需氧量" {
          }
          frame "流速", "水位", "瞬时流量" {
          }
        }
        n184 = global read "系统设置全局变量.vi" "首页跳转运维调试"() -> (w786:cluster{"主画面菜单":i32, "运维调试菜单":i32})
        n185 = Bundle By Name(cluster=w786, "主画面菜单"=w783, "运维调试菜单"=w781) -> (w784:cluster{"主画面菜单":i32, "运维调试菜单":i32})
        n186 = Send Notification(notification=w783, notifier=w785) -> ()  [unwired: 1 in, 2 out]
        n187 = Send Notification(notification=w781, notifier=w782) -> ()  [unwired: 1 in, 2 out]
        n188 = global write "系统设置全局变量.vi" "首页跳转运维调试"(w784) -> ()
      }
    }
  }
